vi "CalcSNS_Persona.vi"(10 "Ref Sensor 2":dbl, 11 "Ref Sensor":dbl) -> (3 "delta SNS":dbl)   [LabVIEW 2015]
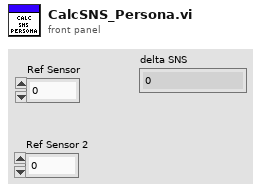
[diagram p1: front panel]
types:
  T1 = cluster{"SNS":dbl, "delta SNS":dbl, "zero SNS":dbl}
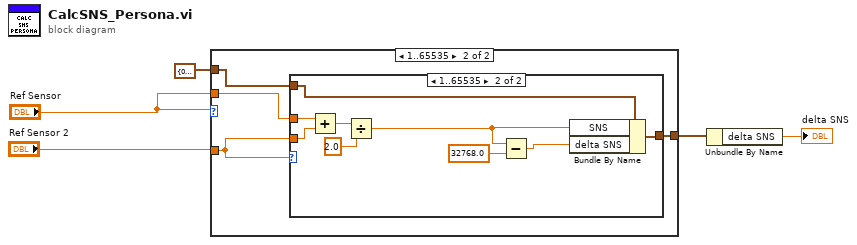
[diagram p0: block diagram]
diagram:
  n1 = case shown="1..65535" "Ref Sensor" {
    tunnel: "Ref Sensor" -> [_ w10]
    tunnel: "Ref Sensor 2" -> [_ w7]
    tunnel: [w6 w9] -> w4
    tunnel: T1 {"SNS"=0.0, "delta SNS"=0.0, "zero SNS"=0.0} ("SNS") -> [w6 w8]
    frame 0, Default {
    }
    frame 1..65535 {
      n2 = case shown="1..65535" w7 {
        tunnel: w7 -> [_ w19]
        tunnel: w10 -> [_ w17]
        tunnel: [w11 w15] -> w9
        tunnel: w8 -> [w11 w14]
        frame 0, Default {
        }
        frame 1..65535 {
          n3 = Add(x=w17, y=w19) -> (x+y=w20:dbl)
          n4 = Divide(x=w20, y=2.0) -> (x/y=w13:dbl)
          n5 = Subtract(x=w13, y=32768.0) -> (x-y=w16:dbl)
          n6 = Bundle By Name(cluster=w14, "SNS"=w13, "delta SNS"=w16) -> (w15:T1)
        }
      }
    }
  }
  n7 = Unbundle By Name(w4) -> ("delta SNS"=→"delta SNS":dbl)
